vi "GenPulseTrain.vi"(4 "duty cycle (0.5)":dbl=0.5 format="%.6f", 5 "gate mode (ungated:0)":T2(ring), 6 "frequency (Hz)":dbl=1.0 format="%.6f", 7 "pulse polarity (high:0)":enum16{"high pulse ", "low pulse"}(ring), 8 "delay":dbl format="%.2f", 9 "number of pulses (cont:0)":i32, 10 "counter":string="1", 11 "device":i16=1) -> (1 "actual parameters":T1 {"pulse width" format="%.6f"; "pulse delay" format="%.6f"; "duty cycle" format="%.6f"; "frequency" format="%.6f"}, 2 "[taskID of counter-1]":u32 format="%.0x", 3 "[taskID of counter]":u32 format="%.0x")   [LabVIEW 2022 SP3]
doc: "Configures the specified counter to generate a continuous pulse-train on the counter's OUT pin, or to generate a finite-length pulse-train using the specified counter and an adjacent counter."
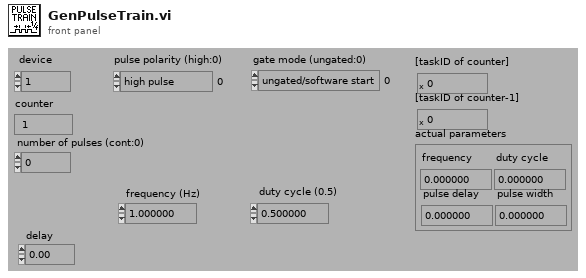
[diagram p1: front panel]
types:
  T1 = cluster{"frequency":dbl, "duty cycle":dbl, "pulse delay":dbl, "pulse width":dbl}
  T2 = enum16{"ungated/software start", "count while high", "count while low", "start on rising edge", "start on falling edge"}
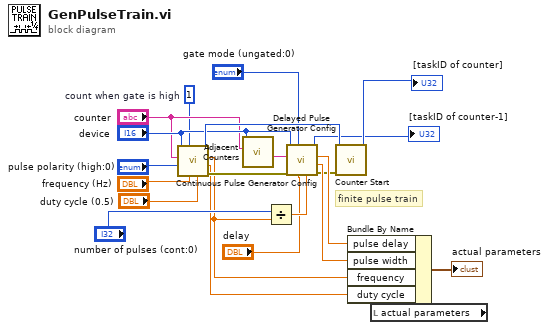
[diagram p0: block diagram]
diagram:
  w13 = u16 1  # count when gate is high
  # "finite pulse train"
  n1 = call <vilib>:"Continuous Pulse Generator Config.vi"("duty cycle (0.5)"="duty cycle (0.5)", "frequency (Hz)"="frequency (Hz)", "gate mode (ungated:0)"=w13, "pulse polarity (high:0)"="pulse polarity (high:0)", "counter"="counter", "device"="device") -> ("error out"=w20:errorcluster, "[actual duty cycle]"=w12:dbl, "[actual frequency (Hz)]"=w9:dbl, "taskID"=w21:u32)  [unwired: 2 in]
  n2 = call <vilib>:"Adjacent Counters.vi"("counter (\"1\")"="counter", "device"="device") -> ("counter-1"=w4:string)  [unwired: 2 in, 7 out]
  n3 = Divide(x="number of pulses (cont:0)", y=w9) -> (x/y=w5:dbl)
  n4 = call <vilib>:"Delayed Pulse Generator Config.vi"("pulse width (s or cycles)"=w5, "pulse delay (s or cycles)"="delay", "gate mode (ungated:0)"="gate mode (ungated:0)", "error in (no error)"=w20, "counter"=w4, "device"="device") -> ("error out"=w6:errorcluster, "[actual width (s or cycles)]"=w8:dbl, "[actual delay (s or cycles)]"=w7:dbl, "taskID"=→"[taskID of counter-1]":u32)  [unwired: 2 in]
  n5 = call <vilib>:"Counter Start.vi"("error in (no error)"=w6, "taskID"=w21) -> ("taskID"=→"[taskID of counter]":u32)  [unwired: 8 in, 1 out]
  n6 = local read "actual parameters"() -> (w10:T1)
  n7 = Bundle By Name(cluster=w10, "pulse delay"=w7, "pulse width"=w8, "frequency"=w9, "duty cycle"=w12) -> (→"actual parameters":T1)
